vi "disableServosArduinoNew.vi"(0 "delay (ms)":u32) -> ()   [LabVIEW 2012]
uses:
  GlobalArduinoNew.vi
  <vilib>/LabVIEW Interface for Arduino/LabVIEW Interface for Arduino.lvlib
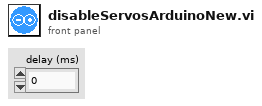
[diagram p1: front panel]
types:
  T1 = typedef "LabVIEW Interface for Arduino.lvlib/Arduino Resource.ctl" = cluster{"VISA resource":refnum<visa-resource-name>, "Board Type":T2, "Connection Type":enum8{"USB / Serial"}, "Bytes Per Packet (15)":u8}
  T2 = typedef "LabVIEW Interface for Arduino.lvlib/Board Type.ctl" = enum16{"Uno", "Dimuelanove w/Atmega 328", "Mega 2560"}
  T3 = typedef "Semaphore RefNum" = refnum<k1>
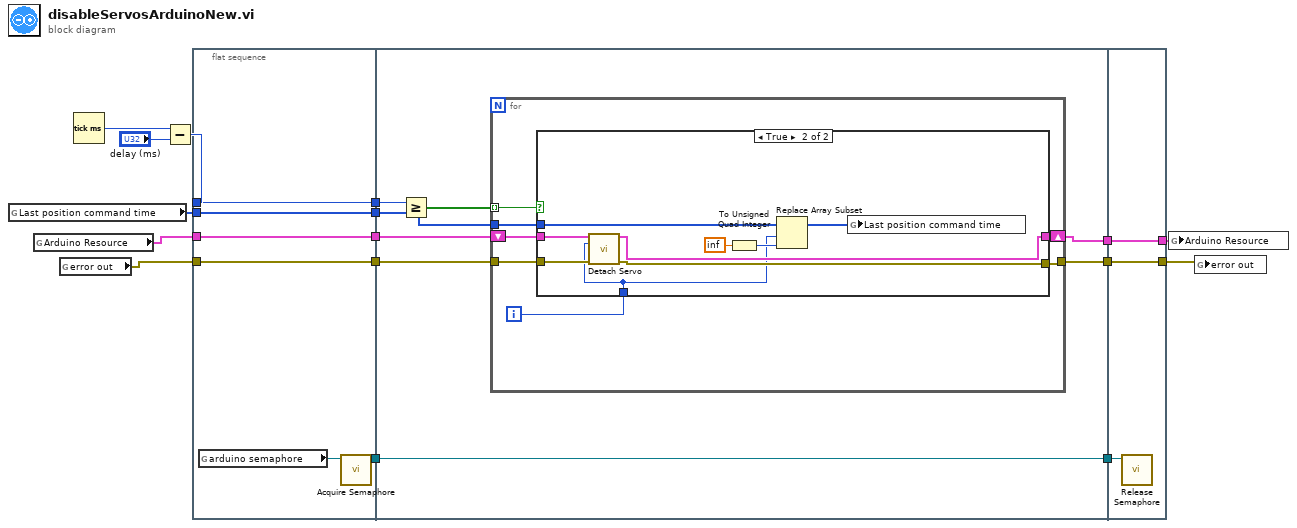
[diagram p0: block diagram]
diagram:
  n1 = global read "GlobalArduinoNew.vi" "Last position command time"() -> (w13:u64[])
  n2 = global read "GlobalArduinoNew.vi" "Arduino Resource"() -> (w12:T1)
  n3 = global read "GlobalArduinoNew.vi" "error out"() -> (w11:errorcluster)
  n4 = Tick Count (ms)() -> (millisecond timer value=w16:u32)
  n5 = Subtract(x=w16, y="delay (ms)") -> (x-y=w14:u32)
  n6 = flat-sequence {
    tunnel: w11 -> [w19]
    tunnel: w12 -> [w20]
    tunnel: w13 -> [w21]
    tunnel: w14 -> [w22]
    tunnel: [w22] -> w8
    tunnel: [w21] -> w7
    tunnel: [w20] -> w6
    tunnel: [w19] -> w5
    tunnel: [w17] -> w2
    tunnel: w8 -> [w30]
    tunnel: w7 -> [w28]
    tunnel: w6 -> [w27]
    tunnel: w5 -> [w26]
    tunnel: [w25] -> w4
    tunnel: [w24] -> w3
    tunnel: w2 -> [w23]
    tunnel: [w23] -> w1
    tunnel: [w50] -> w9
    tunnel: [w51] -> w10
    tunnel: w4 -> [w51]
    tunnel: w3 -> [w50]
    tunnel: w1 -> [w49]
    frame #0 {
      n7 = global read "GlobalArduinoNew.vi" "arduino semaphore"() -> (w18:T3)
      n8 = call <vilib>:"Acquire Semaphore.vi"("semaphore"=w18) -> ("semaphore out"=w17:T3)  [unwired: 4 in, 2 out]
    }
    frame #1 {
      n9 = Greater Or Equal?(x=w30, y=w28) -> (x >= y?=w29:bool[])
      n10 = for {
        tunnel: w29 -> [w37] mode=indexing
        tunnel: w28 -> [w35]
        shift-right: [w33] -> w25
        shift-left: w27 -> [w34]
        tunnel: w26 -> [w32]
        tunnel: [w31] -> w24
        i -> [w36]
        n11 = case shown="True" w37 {
          tunnel: w36 -> [_ w40]
          tunnel: w35 -> [_ w48]
          tunnel: w34 -> [w39 w44]
          tunnel: [w39 w43] -> w33
          tunnel: w32 -> [w38 w42]
          tunnel: [w38 w41] -> w31
          frame False {
          }
          frame True {
            n12 = call <vilib>:"Detach Servo.vi"("Arduino Resource"=w44, "Servo Number"=w40, "error in"=w42) -> ("Arduino Resource"=w43:T1, "error out"=w41:errorcluster)  [unwired: 11 in]
            n13 = To Unsigned Quad Integer(1:inf) -> (0:w46:u64)
            n14 = Replace Array Subset(array=w48, new element=w46, index=w40) -> (w45:u64[])
            n15 = global write "GlobalArduinoNew.vi" "Last position command time"(w45) -> ()
          }
        }
      }
    }
    frame #2 {
      n16 = call <vilib>:"Release Semaphore.vi"("semaphore"=w49) -> ()  [unwired: 5 in, 2 out]
    }
  }
  n17 = global write "GlobalArduinoNew.vi" "Arduino Resource"(w10) -> ()
  n18 = global write "GlobalArduinoNew.vi" "error out"(w9) -> ()
